vi "New.vi"(8 "error in (no error)":errorcluster, 11 "reference in":refnum<class "[Test Suite] File Transfer Behavior.lvclass">) -> (0 "error out":errorcluster, 3 "reference out":refnum<class "[Test Suite] File Transfer Behavior.lvclass">)   [LabVIEW 2015, in "Tests.lvlib" / "[Test Suite] File Transfer Behavior.lvclass"]
uses:
  [Test Suite] File Transfer Behavior.lvclass
  <vilib>/addons/_JKI Toolkits/VI Tester/TestCase.llb/TestCase.lvclass
  [Test Suite] File Transfer Behavior.lvclass/[Test Suite] File Transfer Behavior.ctl
  <vilib>/addons/_JKI Toolkits/VI Tester/TestSuite.llb/TestSuite.lvclass
panel:
  in  "Targets":T1(array[cluster])
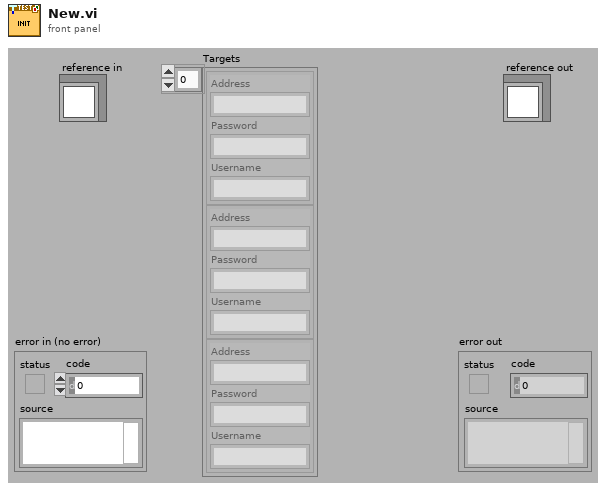
[diagram p1: front panel]
types:
  T1 = cluster{"Address":string, "Password":string, "Username":string}[]
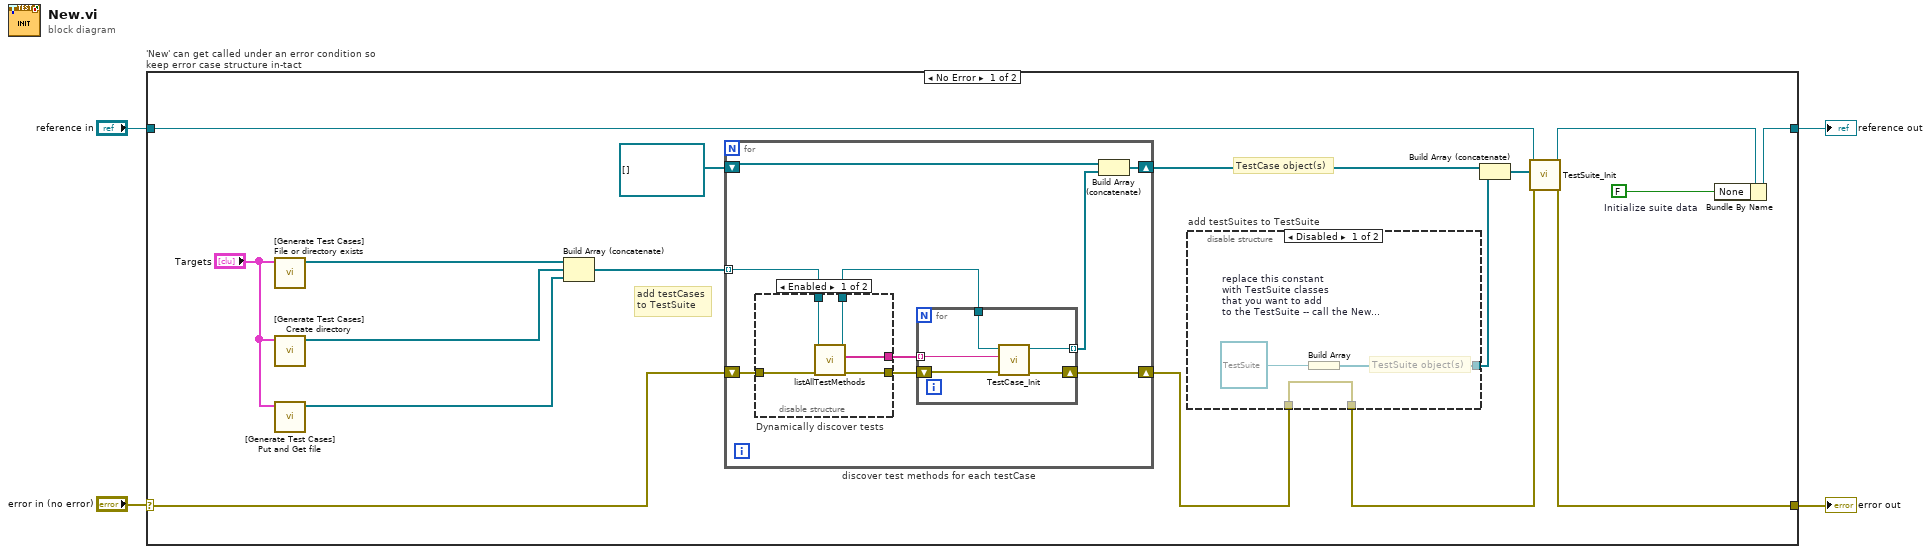
[diagram p0: block diagram]
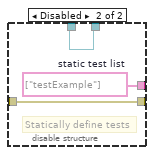
[diagram p2: hidden frame]
diagram:
  n1 = case "'New' can get called under an error condition so keep error case structure in-tact" shown="No Error" "error in (no error)" {
    selector: "error in (no error)" -> [w16 w48]
    tunnel: [w21 w49] -> w4
    tunnel: "reference in" -> [w17 w49]
    tunnel: [w18 w48] -> w1
    frame No Error {
      w20 = FALSE  # Initialize suite data
      # "TestCase object(s)"
      # "add testCases to TestSuite"
      n2 = call "[Generate Test Cases] File or directory exists.vi"("Targets"="Targets") -> ("Test Cases"=w9:refnum<class "TestCase.lvclass">[])  [unwired: 10 in]
      n3 = call "[Generate Test Cases] Create directory.vi"("Targets"="Targets") -> ("Test Cases"=w7:refnum<class "TestCase.lvclass">[])  [unwired: 10 in]
      n4 = call "[Generate Test Cases] Put and Get file.vi"("Targets"="Targets") -> ("Test Cases"=w6:refnum<class "TestCase.lvclass">[])  [unwired: 10 in]
      n5 = Build Array (concatenate)(w9, w7, w6) -> (w8:refnum<class "TestCase.lvclass">[])
      n6 = for "discover test methods for each testCase" {
        shift-right: [w30] -> w11
        shift-left: w16 -> [w26]
        tunnel: w8 -> [w23] mode=indexing
        shift-right: [w27] -> w15
        shift-left: refnum<class "TestCase.lvclass">[] [] -> [w28]
        n7 = disable-structure "Dynamically discover tests" shown="Enabled" {
          disable-tunnel: w26 -> [w35 w36]
          disable-tunnel: [w34 w36] -> w25
          disable-tunnel: [w33 w37] -> w24
          disable-tunnel: w23 -> [w32 w38]
          disable-tunnel: [w31 w38] -> w22
          frame Enabled {
            n8 = call-dynamic "listAllTestMethods.vi"("error in (no error)"=w35, "TestCase in"=w32) -> ("error out"=w34:errorcluster, "test methods"=w33:string[], "TestCase out"=w31:refnum<class "TestCase.lvclass">)  [unwired: 7 in]
          }
          frame Disabled {
            w37 = string[] ["testExample"]  # static test list
            # "Statically define tests"
          }
        }
        n9 = for {
          tunnel: w22 -> [w39]
          tunnel: w24 -> [w43] mode=indexing
          shift-right: [w41] -> w30
          shift-left: w25 -> [w42]
          tunnel: [w40] -> w29 mode=indexing
          n10 = call <vilib>:"TestCase_Init.vi"("error in (no error)"=w42, "methodName (\"runTest\")"=w43, "TestCase in"=w39) -> ("error out"=w41:errorcluster, "TestCase out"=w40:refnum<class "TestCase.lvclass">)  [unwired: 7 in]
        }
        n11 = Build Array (concatenate)(w28, w29) -> (w27:refnum<class "TestCase.lvclass">[])
      }
      n12 = disable-structure "add testSuites to TestSuite" shown="Disabled" {
        disable-tunnel: [w44 _] -> w13
        disable-tunnel: [w46 w47] -> w12
        disable-tunnel: w11 -> [w46 w47]
        frame Disabled {
          w45 = refnum<class "TestSuite.lvclass"> refnum  # replace this constant with TestSuite classes that you want to add to the TestSuite -- call the New method for each TestSuite prior to adding it to this TestSuite
          # "TestSuite object(s)"
          n13 = Build Array(w45) -> (w44:refnum<class "TestSuite.lvclass">[])
        }
        frame Enabled {
          # "by default, no TestSuites are defined\nas members of a TestSuite"
        }
      }
      n14 = Build Array (concatenate)(w15, w13) -> (w14:refnum<class>[])
      n15 = call <vilib>:"TestSuite_Init.vi"("error in (no error)"=w12, "tests (none)"=w14, "TestSuite in"=w17) -> ("error out"=w18:errorcluster, "TestSuite out"=w19:refnum<class "[Test Suite] File Transfer Behavior.lvclass">)  [unwired: 7 in]
      n16 = Bundle By Name(cluster=w19, "None"=w20) -> (w21:refnum<class "[Test Suite] File Transfer Behavior.lvclass">)
    }
    frame Error {
    }
  }
  "reference out" <- w4
  "error out" <- w1
